vi "SampleRateknob.vi"(0 "Dial":u32(knob) scale=0.0..29.0, 3 "error in (no error)":errorcluster) -> (5 "Sampling Rate":dbl format="%.2e", 8 "error out":errorcluster)   [LabVIEW 2014]
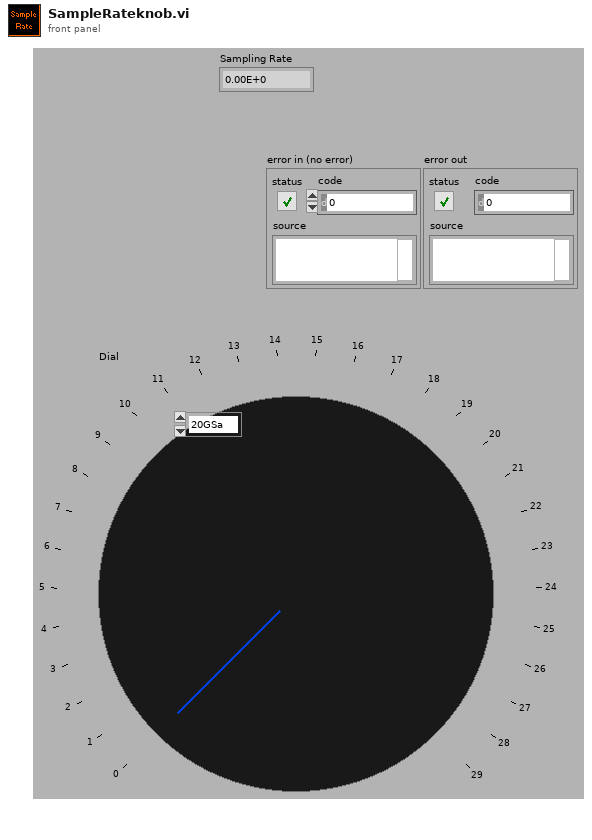
[diagram p1: front panel]
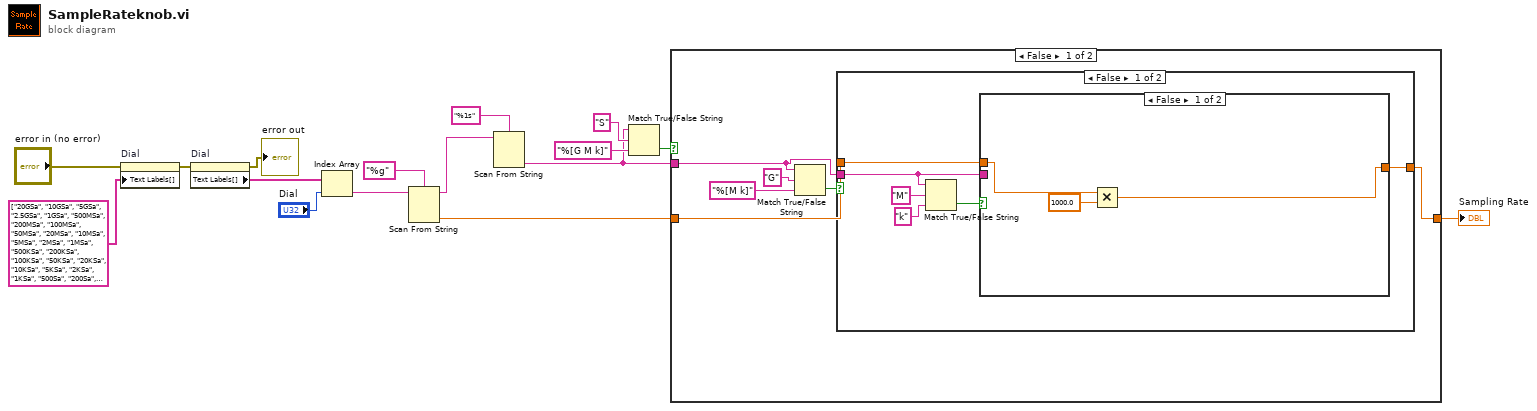
[diagram p0: block diagram]
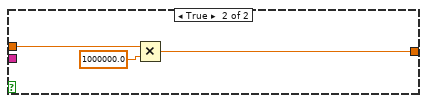
[diagram p2: hidden frame]
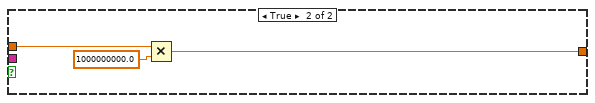
[diagram p3: hidden frame]
diagram:
  n1 = property on="Dial" class="Knob (strict)"(error in="error in (no error)", "Text Labels[]"=string[] ["20GSa", "10GSa", "5GSa", "2.5GSa", "1GSa", "500MSa", "200MSa", "100MSa", "50MSa", "20MSa", "10MSa", "5MSa", "2MSa", "1MSa", "500KSa", "200KSa", "100KSa", "50KSa", "20KSa", "10KSa", "5KSa", "2KSa", "1KSa", "500Sa", "200Sa", "100Sa", "50Sa", "20Sa", "10Sa", "5Sa"]) -> (error out=w12:errorcluster)  [unwired: 1 in, 1 out]
  n2 = property on="Dial" class="Knob (strict)"(error in=w12) -> (error out=→"error out":errorcluster, "Text Labels[]"=w13:string[])  [unwired: 1 in, 1 out]
  n3 = Index Array(array=w13, index="Dial") -> (element=w1:string)
  n4 = Scan From String(format string="%g", input string=w1) -> (remaining string=w10:string, output 1=w4:dbl)  [unwired: 3 in, 2 out]
  n5 = Scan From String(format string="%1s", input string=w10) -> (output 1=w3:string)  [unwired: 3 in, 3 out]
  n6 = Match True/False String(2:"%[G M k]" ("false string"), 3:"S" ("true string"), 4:w3) -> (0:w7:bool)  [unwired: 1 out]
  n7 = case shown="False" w7 {
    tunnel: w4 -> [w19 w38]
    tunnel: [w17 w38] -> w2
    tunnel: w3 -> [w18 _]
    frame False {
      n8 = Match True/False String(2:"%[M k]" ("false string"), 3:"G" ("true string"), 4:w18) -> (0:w21:bool)  [unwired: 1 out]
      n9 = case shown="False" w21 {
        tunnel: w19 -> [w25 w37]
        tunnel: [w24 w35] -> w17
        tunnel: w18 -> [w23 _]
        frame False {
          n10 = Match True/False String(2:"k" ("false string"), 3:"M" ("true string"), 4:w23) -> (0:w28:bool)  [unwired: 1 out]
          n11 = case shown="False" w28 {
            tunnel: w25 -> [w31 w34]
            tunnel: [w29 w32] -> w24
            tunnel: w23 -> [_ _]
            frame False {
              n12 = Multiply(x=w31, y=1000.0) -> (x*y=w29:dbl)
            }
            frame True {
              n13 = Multiply(x=w34, y=1000000.0) -> (x*y=w32:dbl)
            }
          }
        }
        frame True {
          n14 = Multiply(x=w37, y=1000000000.0) -> (x*y=w35:dbl)
        }
      }
    }
    frame True {
    }
  }
  "Sampling Rate" <- w2
